vi "Build Repeat Event.vi"(8 "error in (no error)":errorcluster, 10 "Event":T1) -> (0 "error out":errorcluster, 3 "New Event Msg out":refnum<class "New Event Msg.lvclass">)   [LabVIEW 2019, in "Controller.lvlib" / "New Event Msg.lvclass"]
uses:
  New Event Msg.lvclass
  Sensors/Detector/Event.ctl
  Sensors/Detector/Muon Detector.lvclass
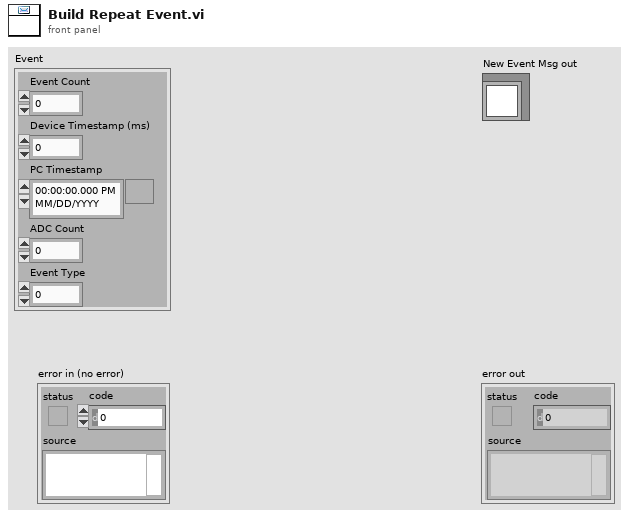
[diagram p1: front panel]
types:
  T1 = typedef "Muon Detector.lvclass/Event.ctl" = cluster{"Event Count":i32, "Device Timestamp (ms)":i32, "PC Timestamp":timestamp, "ADC Count":i32, "Event Type":u8}
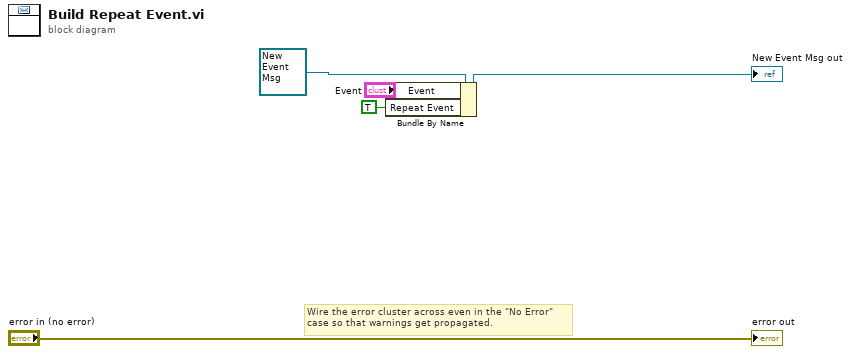
[diagram p0: block diagram]
diagram:
  # "Wire the error cluster across even in the \"No Error\"\ncase so that warnings get propagated."
  n1 = Bundle By Name(cluster=refnum<class "New Event Msg.lvclass"> refnum ("New Event Msg in"), "Event"="Event", "Repeat Event"=TRUE) -> (→"New Event Msg out":refnum<class "New Event Msg.lvclass">)
  "error out" <- "error in (no error)"
